vi "Cannon Arming.vi"(1 "Cannon Info In":T2) -> (0 "Cannon Info Out":T2)   [LabVIEW 2013]
uses:
  <vilib>/Rock Robotics/WPI/Relay/WPI_RelayValue.ctl
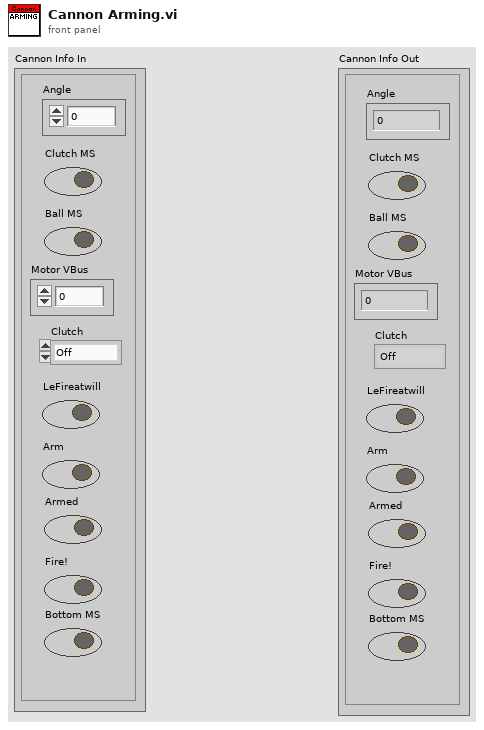
[diagram p1: front panel]
types:
  T1 = typedef "WPI_RelayValue.ctl" = enum16{"Off", "On", "Forward", "Reverse"}
  T2 = cluster{"Angle":dbl, "Clutch MS":bool, "Ball MS":bool, "Clutch ":T1, "LeFireatwill":bool, "Arm":bool, "Armed":bool, "Fire!":bool, "Bottom MS":bool, "Motor VBus":dbl}
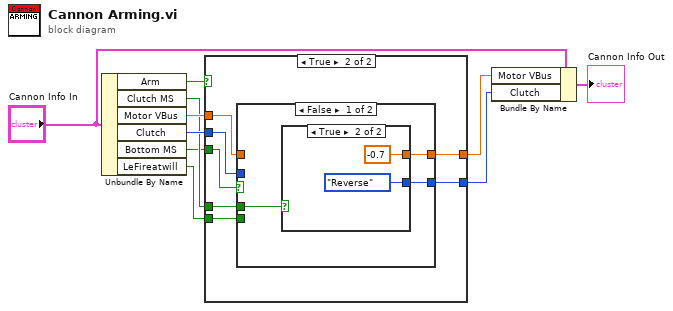
[diagram p0: block diagram]
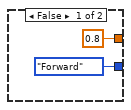
[diagram p3: hidden frame]
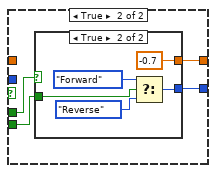
[diagram p4: hidden frame]
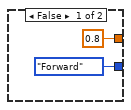
[diagram p5: hidden frame]
diagram:
  n1 = Unbundle By Name("Cannon Info In") -> ("Arm"=w1:bool, "Clutch MS"=w6:bool, "Motor VBus"=w10:dbl, "Clutch"=w9:T1, "Bottom MS"=w5:bool, "LeFireatwill"=w4:bool)
  n2 = case shown="True" w1 {
    tunnel: w10 -> [w12 w19]
    tunnel: w9 -> [w11 w18]
    tunnel: [w12 w17] -> w8
    tunnel: [w11 w16] -> w7
    tunnel: w6 -> [_ w15]
    tunnel: w5 -> [_ w14]
    tunnel: w4 -> [_ w13]
    frame False {
    }
    frame True {
      n3 = case shown="False" w14 {
        tunnel: w15 -> [w22 w30]
        tunnel: w19 -> [_ _]
        tunnel: [w21 w29] -> w17
        tunnel: [w20 w28] -> w16
        tunnel: w18 -> [_ _]
        tunnel: w13 -> [_ w27]
        frame False {
          n4 = case shown="True" w22 {
            tunnel: [0.8 -0.7] -> w21
            tunnel: [WPI_RelayValue."Forward" ("Clutch") WPI_RelayValue."Reverse" ("Clutch")] -> w20
            frame False {
            }
            frame True {
            }
          }
        }
        frame True {
          n5 = case shown="True" w30 {
            tunnel: [0.8 -0.7] -> w29
            tunnel: [WPI_RelayValue."Forward" ("Clutch") w33] -> w28
            tunnel: w27 -> [_ w36]
            frame False {
            }
            frame True {
              n6 = Select(t=WPI_RelayValue."Forward", s=w36, f=WPI_RelayValue."Reverse" ("Clutch")) -> (s? t:f=w33:T1)
            }
          }
        }
      }
    }
  }
  n7 = Bundle By Name(cluster="Cannon Info In", "Motor VBus"=w8, "Clutch"=w7) -> (→"Cannon Info Out":T2)
